vi "DSF.Engine.Buffer Converter.Set Data Type Buffers.vi"(10 "data type buffers":T1, 11 "Buffer Converter in":refnum<class "Buffer Converter.lvclass">) -> (3 "Buffer Converter out":refnum<class "Buffer Converter.lvclass">)   [LabVIEW 2017, in "Data Sharing Framework Engine.lvlib" / "Buffer Converter.lvclass"]
uses:
  Buffer Converter.lvclass
  Shared/Typedefs/DSF Runtime Type Buffers.ctl
  Buffer Converter.lvclass/Buffer Converter.ctl
  Source/Data Sharing Framework Core/Engine/Data Sharing Framework Engine.lvlib
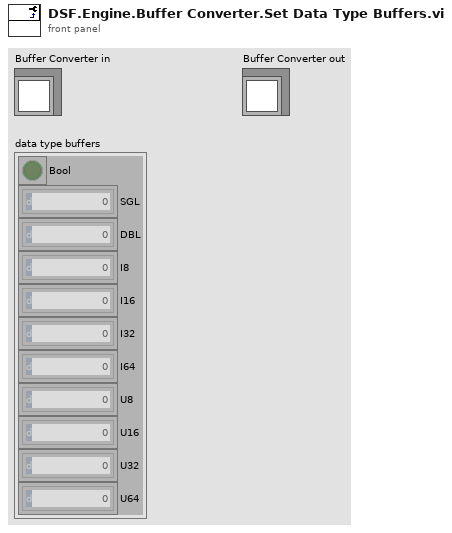
[diagram p1: front panel]
types:
  T1 = typedef "Data Sharing Framework Engine.lvlib/DSF Runtime Type Buffers.ctl" = cluster{"Bool":bool[], "SGL":sgl[], "DBL":dbl[], "I8":i8[], "I16":i16[], "I32":i32[], "I64":i64[], "U8":u8[], "U16":u16[], "U32":u32[], "U64":u64[]}
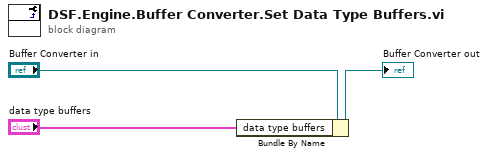
[diagram p0: block diagram]
diagram:
  n1 = Bundle By Name(cluster="Buffer Converter in", "data type buffers"="data type buffers") -> (→"Buffer Converter out":refnum<class "Buffer Converter.lvclass">)
